vi "ThermiToTemp.vi"(8 "γ":dbl=1.018703e-07 format="%#_6e", 9 "β":dbl=0.0002343159 format="%#_6e", 10 "α":dbl=0.00129536 format="%#_6e", 11 "Rt":dbl) -> (0 "Tc":dbl, 3 "Tk":dbl)   [LabVIEW 2012]
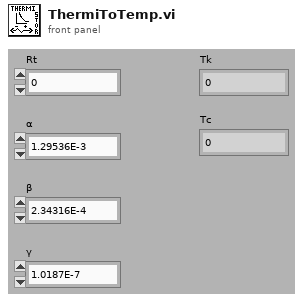
[diagram p1: front panel]
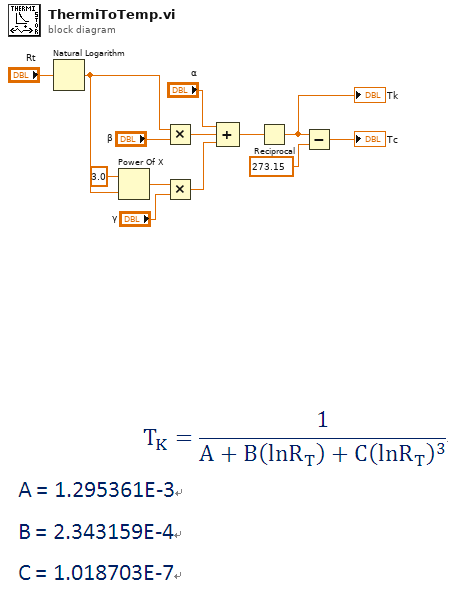
[diagram p0: block diagram]
diagram:
  n1 = Natural Logarithm(1:"Rt") -> (0:w11:dbl)
  n2 = Power Of X(1:w11, 2:3.0 ("y")) -> (0:w9:dbl)
  n3 = Multiply(x=w11, y="β") -> (x*y=w6:dbl)
  n4 = Multiply(x=w9, y="γ") -> (x*y=w5:dbl)
  n5 = Compound Arithmetic op=ADD("α", w6, w5) -> (w4:dbl)
  n6 = Reciprocal(x=w4) -> (1/x=w3:dbl)
  "Tk" <- w3
  n7 = Subtract(x=w3, y=273.15) -> (x-y=→"Tc":dbl)
